vi "Disabled.vi"(7 "Robot Mode":T2, 10 "Match Info":T1={"Autonomous Elapsed Seconds"=0.0, "TeleOp Elapsed Seconds"=0.0, "Disabled Elapsed Seconds"=0.0, "Visited Autonomous"=FALSE, "Visited TeleOp"=FALSE, "Visited Disabled"=FALSE, "Autonomous Settings"={"Autonomous Style"=enum."Independent", "VI Refnum"=refnum}}, 11 "Call Context":T3) -> ()   [LabVIEW 2012]
doc: "This VI is called each time a disabled packet is received from the DS. It is often used to prepare for the next robot mode, to calibrate sensors, etc."
uses:
  <vilib>/Rock Robotics/WPI/DriverStation/WPI_DriverStationDerivedRobotMode.ctl
  <vilib>/Rock Robotics/WPI/DriverStation/WPI_DriverStationRobotMode2.ctl
  <vilib>/Rock Robotics/WPI/DriverStation/WPI_DriverStationMatch Info.ctl
  Systems/Drive/Or David (Drive Global Data).vi
  Systems/Conveyer Belt/Conveyer Belt Global Data.vi
  Systems/Cannon/Cannon Global Data.vi
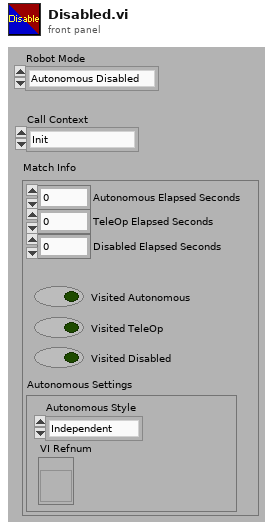
[diagram p1: front panel]
types:
  T1 = typedef "WPI_DriverStationMatch Info.ctl" = cluster{"Autonomous Elapsed Seconds":dbl, "TeleOp Elapsed Seconds":dbl, "Disabled Elapsed Seconds":dbl, "Visited Autonomous":bool, "Visited TeleOp":bool, "Visited Disabled":bool, "Autonomous Settings":cluster{"Autonomous Style":enum16{"Iterative", "Independent"}, "VI Refnum":refnum<vi>}}
  T2 = typedef "WPI_DriverStationRobotMode2.ctl" = enum16{"Autonomous Disabled", "Autonomous Enabled", "Teleop Disabled", "Teleop Enabled", "Timeout", "Finish", "Test Disabled", "Test Enabled"}
  T3 = typedef "WPI_DriverStationDerivedRobotMode.ctl" = enum16{"Init", "Execute", "Stop"}
  T4 = typedef "WPI_SolenoidValue.ctl" = enum16{"Off", "On", "Forward", "Reverse"}
  T5 = cluster{"Shifter?":bool, "Axisses":dbl[], "Shifter Value":T4}
  T6 = cluster{"Throttle":dbl, "RPM":dbl, "Motor VBus":dbl}
  T7 = cluster{"Horizontal Belt":dbl, "Vertical Belt":dbl, "MS":bool}
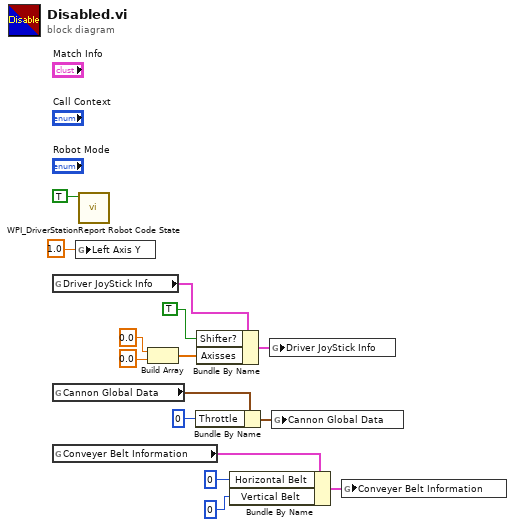
[diagram p0: block diagram]
diagram:
  n1 = global read "Or David (Drive Global Data).vi" "Driver JoyStick Info"() -> (w12:T5)
  n2 = global read "Cannon Global Data.vi" "Cannon Global Data"() -> (w13:T6)
  n3 = global read "Conveyer Belt Global Data.vi" "Conveyer Belt Information"() -> (w9:T7)
  n4 = global write "Or David (Drive Global Data).vi" "Left Axis Y"(1.0 ("Left Axis Y")) -> ()
  n5 = call <vilib>:"WPI_DriverStationReport Robot Code State.vi"("Disabled"=TRUE ("Autonomous")) -> ()  [unwired: 10 in, 1 out]
  n6 = Build Array(0.0, 0.0) -> (w5:dbl[])
  n7 = Bundle By Name(cluster=w13, "Throttle"=0) -> (w14:T6)
  n8 = Bundle By Name(cluster=w12, "Shifter?"=TRUE, "Axisses"=w5) -> (w11:T5)
  n9 = Bundle By Name(cluster=w9, "Horizontal Belt"=0, "Vertical Belt"=0) -> (w10:T7)
  n10 = global write "Or David (Drive Global Data).vi" "Driver JoyStick Info"(w11) -> ()
  n11 = global write "Cannon Global Data.vi" "Cannon Global Data"(w14) -> ()
  n12 = global write "Conveyer Belt Global Data.vi" "Conveyer Belt Information"(w10) -> ()
